vi "getFile.vi"(8 "error in (no error)":errorcluster, 9 "local path":path, 10 "remote path":string, 11 "ConnectionData":T1) -> (0 "error out":errorcluster, 3 "local path out":path)   [LabVIEW 2015]
uses:
  connectionData.ctl
panel:
  # "Gets a file from a remote location. Uses the pscp utility to perform the\ntransfer. This VI expects to find pscp.exe in the same dirctory that\nthis VI is located in.\nDOWNLOAD: http://www.chiark.greenend.org.uk/~sgtatham/putty/download.html"
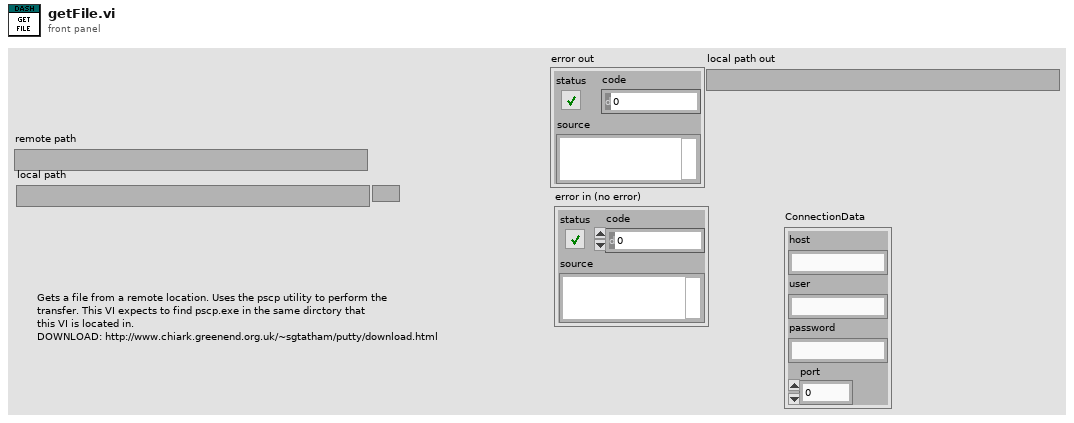
[diagram p1: front panel]
types:
  T1 = typedef "connectionData.ctl" = cluster{"host":string, "user":string, "password":string, "port":u16}
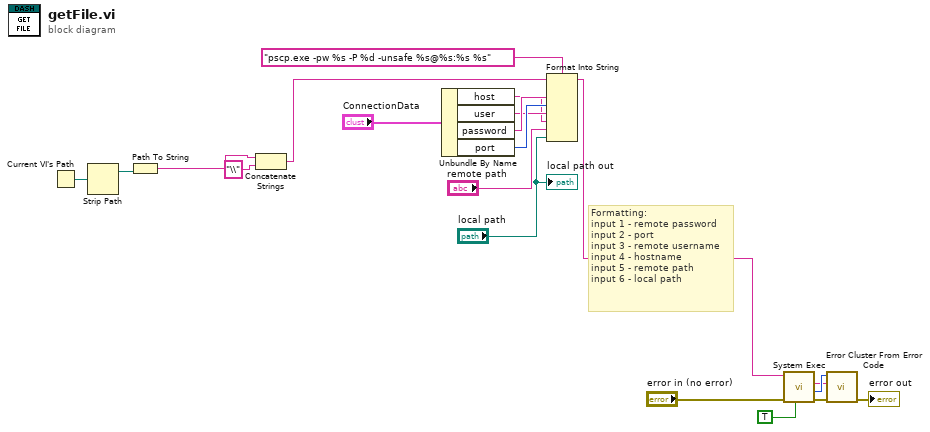
[diagram p0: block diagram]
diagram:
  # "Formatting:\ninput 1 - remote password\ninput 2 - port\ninput 3 - remote username\ninput 4 - hostname\ninput 5 - remote path\ninput 6 - local path"
  n1 = Current VI's Path() -> (path=w5:path)
  n2 = Strip Path(path=w5) -> (stripped path=w3:path)  [unwired: 1 out]
  n3 = Path To String(path=w3) -> (string=w2:string)
  n4 = Concatenate Strings(w2, "\\" ("string")) -> (w1:string)
  n5 = Unbundle By Name("ConnectionData") -> ("host"=w7:string, "user"=w8:string, "password"=w9:string, "port"=w10:u16)
  n6 = Format Into String(format string="pscp.exe -pw %s -P %d -unsafe %s@%s:%s %s", initial string=w1, w9, w10, w8, w7, "remote path", "local path") -> (resulting string=w15:string)  [unwired: 1 in, 1 out]
  n7 = call <vilib>:"System Exec.vi"("run minimized? (F)"=TRUE, "error in (no error)"="error in (no error)", "command line"=w15) -> ("error out"=w17:errorcluster, "return code"=w19:i32, "standard error"=w18:string)  [unwired: 5 in, 1 out]
  n8 = call <vilib>:"Error Cluster From Error Code.vi"("error in (no error)"=w17, "error message (\"\")"=w18, "error code (0)"=w19) -> ("error out"=→"error out":errorcluster)  [unwired: 6 in]
  "local path out" <- "local path"
